vi "Simple Example.vi"() -> ()   [LabVIEW 2020, in "Simple Example.lvlib"]
uses:
  Simple Example.lvlib
  Graphics/Libraries/Raster/Raster.lvlib
  Graphics/Libraries/Raster/Rectangle Dimensions.ctl
  Graphics/Libraries/3D/Camera.ctl
  Graphics/Libraries/3D/3D.lvlib
  Graphics/Libraries/3D/Vector 3D.ctl
  Graphics/Libraries/Utility/Utility.lvlib
  Graphics/Libraries/Raster/UV.ctl
  Graphics/Libraries/3D/Vertex.ctl
  Graphics/Libraries/3D/Triangle.ctl
  7fa56694-391c-4e45-8567-979b4c554bf3.vi
  d55de395-ed50-4187-b237-13a560dfed05.vi
  Graphics/Libraries/Raster/Texture.ctl
  Graphics/Libraries/3D/Material.ctl
panel:
  out "Raaster Time [s]":dbl
  in  "Textured":bool=TRUE
  out "FPS":dbl
  in  "z Transform":sgl(slide)=-15.0 scale=-20.0..10.0
  in  "y Transform":sgl(slide)=5.0 scale=-10.0..10.0
  in  "x Transform":sgl(slide) scale=-10.0..10.0
  in  "z Rotation":sgl(slide) scale=-360.0..360.0
  in  "y Rotation":sgl(slide) scale=-180.0..180.0
  in  "x Rotation":sgl(slide) scale=-360.0..180.0
  out "Screen":picture
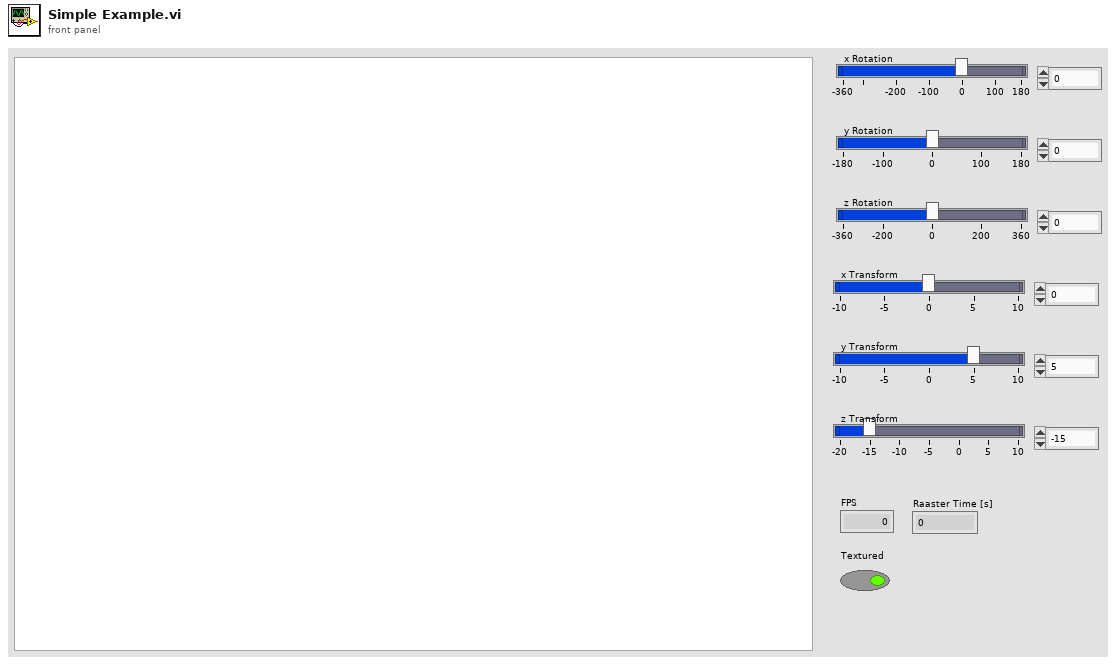
[diagram p1: front panel]
types:
  T1 = typedef "3D.lvlib/Vector 3D.ctl" = cluster{"x":sgl, "y":sgl, "z":sgl}
  T2 = typedef "3D.lvlib/Camera.ctl" = cluster{"Field Of View":sgl, "Near Plane":sgl, "Far Plane":sgl}
  T3 = typedef "Raster.lvlib/Rectangle Dimensions.ctl" = cluster{"Width":u32, "Height":u32}
  T4 = typedef "3D.lvlib/Object.ctl" = cluster{"Triangles":T5[], "Transform":T10, "Name":string, "Alpha Blending Enabled":bool, "Alpha":dbl, "Turntable Enabled":bool, "Material":T8}
  T5 = typedef "3D.lvlib/Triangle.ctl" = cluster{"Vertex 1":T6, "Vertex 2":T6, "Vertex 3":T6, "Alpha":dbl, "Alpha Blending Enabled":bool, "Colour":u32, "Material":T8}
  T6 = typedef "3D.lvlib/Vertex.ctl" = cluster{"Position":T1, "UV":T7, "Colour":u32}
  T7 = typedef "Raster.lvlib/UV.ctl" = cluster{"u":sgl, "v":sgl}
  T8 = typedef "3D.lvlib/Material.ctl" = cluster{"Diffuse Colour":u32, "Texture":T9}
  T9 = typedef "Raster.lvlib/Texture.ctl" = cluster{"Pixels":refnum<data-value>, "Size":T3}
  T10 = typedef "3D.lvlib/Transform.ctl" = cluster{"Position":T1, "Rotation":T1, "Scale":T1}
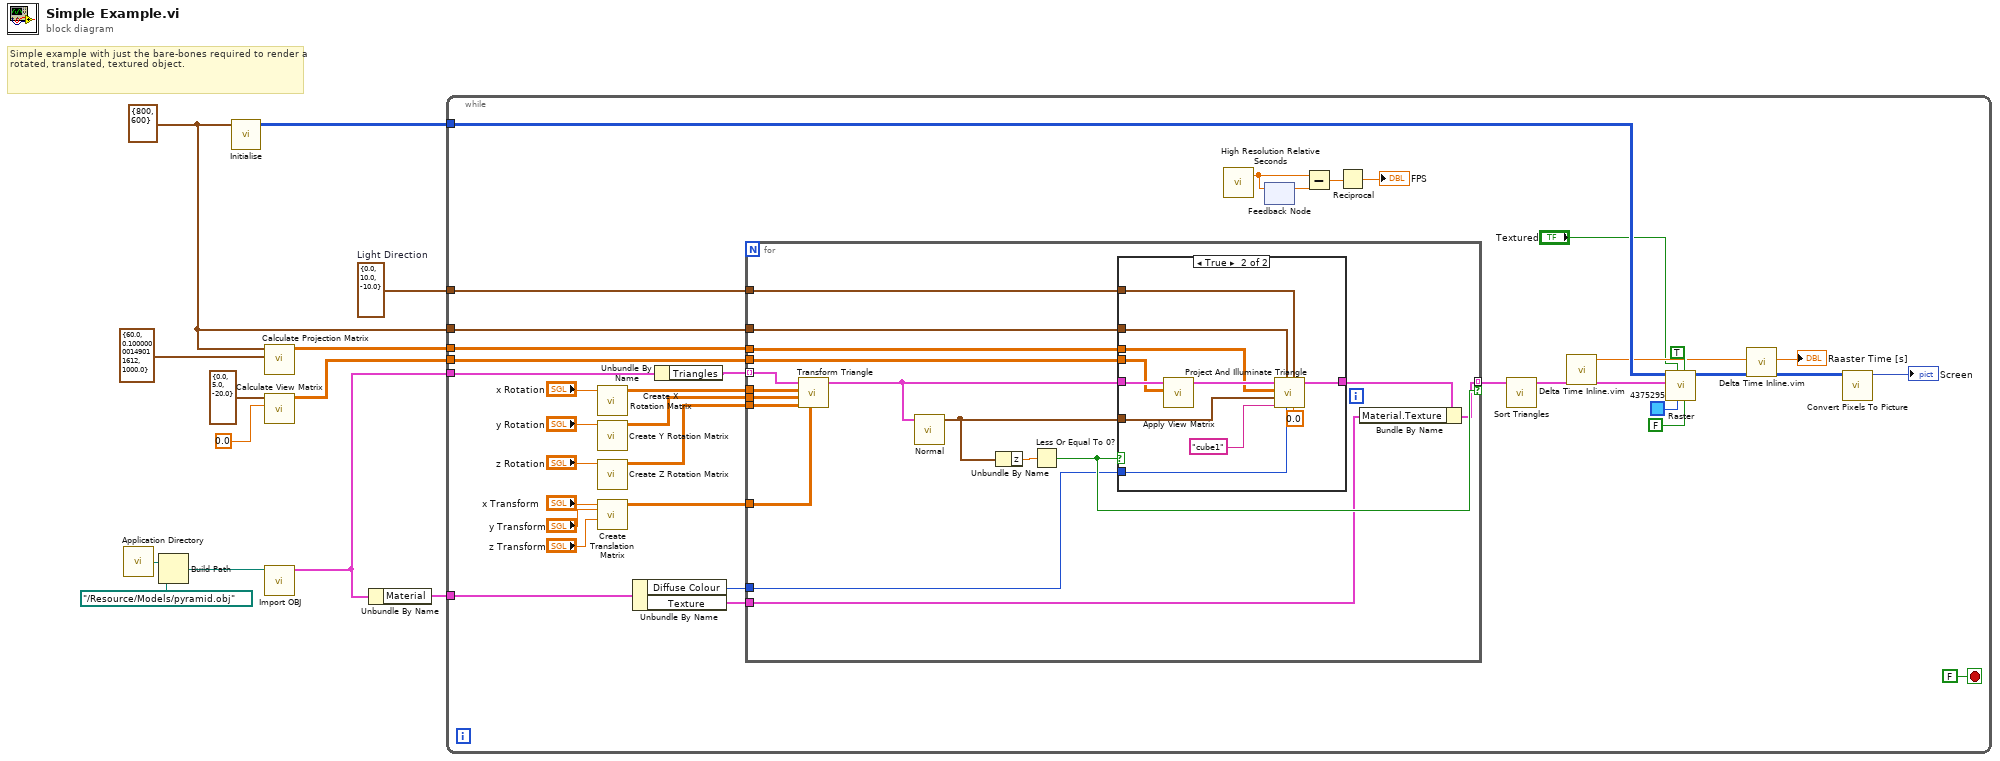
[diagram p0: block diagram]
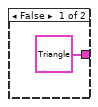
[diagram p2: hidden frame]
diagram:
  w11 = T1 {"x"=0.0, "y"=10.0, "z"=-10.0}  # Light Direction
  w9 = T3 {"Width"=800, "Height"=600} ("Screen Dimensions")
  # "Simple example with just the bare-bones required to render a rotated, translated, textured object."
  n1 = call <vilib>:"Application Directory.vi"() -> ("Application Directory"=w4:path)
  n2 = Build Path(base path=w4, name or relative path=path "../Resource/Models/pyramid.obj") -> (appended path=w3:path)
  n3 = call "Initialise.vi"("Screen Dimensions"=w9) -> ("Pixel Data out"=w8:u32[][])  [unwired: 10 in]
  n4 = call "Calculate Projection Matrix.vi"("Camera"=T2 {"Field Of View"=60.0, "Near Plane"=0.1, "Far Plane"=1000.0}, "Screen Dimensions"=w9) -> ("Projection Matrix"=w10:sgl[][])  [unwired: 9 in]
  n5 = call "Calculate View Matrix.vi"("Camera Rotation"=sgl 0.0, "Camera Position"=T1 {"x"=0.0, "y"=5.0, "z"=-20.0} ("output cluster")) -> ("View Matrix"=w12:sgl[][])  [unwired: 9 in]
  n6 = call "Import OBJ.vi"("Object"=w3) -> ("Object"=w2:T4)  [unwired: 9 in, 1 out]
  n7 = Unbundle By Name(w2) -> ("Material"=w1:T8)
  n8 = while {
    tunnel: w12 -> [w40]
    tunnel: w11 -> [w39]
    tunnel: w10 -> [w38]
    tunnel: w9 -> [w37]
    tunnel: w2 -> [w25]
    tunnel: w8 -> [w36]
    tunnel: w1 -> [w16]
    stop <- FALSE stop-if-true
    n9 = call "Create X Rotation Matrix.vi"("Theta (°)"="x Rotation") -> ("Rotation X Matrix"=w44:sgl[][])  [unwired: 10 in]
    n10 = call "Create Y Rotation Matrix.vi"("Theta (°)"="y Rotation") -> ("Rotation Y Matrix"=w43:sgl[][])  [unwired: 10 in]
    n11 = call "Create Z Rotation Matrix.vi"("Theta (°)"="z Rotation") -> ("Rotation Z Matrix"=w42:sgl[][])  [unwired: 10 in]
    n12 = call "Create Translation Matrix.vi"("z"="z Transform", "y"="y Transform", "x"="x Transform") -> ("Translation Matrix"=w41:sgl[][])  [unwired: 8 in]
    n13 = Unbundle By Name(w16) -> ("Diffuse Colour"=w15:u32, "Texture"=w14:T9)
    n14 = Unbundle By Name(w25) -> ("Triangles"=w26:T5[])
    n15 = for {
      tunnel: w42 -> [w64]
      tunnel: w44 -> [w66]
      tunnel: [w52] -> w24 mode=indexing if=w58
      tunnel: w43 -> [w65]
      tunnel: w41 -> [w63]
      tunnel: w26 -> [w55] mode=indexing
      tunnel: w37 -> [w61]
      tunnel: w38 -> [w60]
      tunnel: w39 -> [w59]
      tunnel: w40 -> [w56]
      tunnel: w15 -> [w54]
      tunnel: w14 -> [w51]
      n16 = call "Transform Triangle.vi"("Translation Matrix"=w63, "Rotation Z Matrix"=w64, "Rotation Y Matrix"=w65, "Rotation X Matrix"=w66, "Triangle in"=w55) -> ("Triangle out"=w62:T5)  [unwired: 6 in]
      n17 = call "Normal.vi"("Triangle"=w62) -> ("Normal"=w67:T1)  [unwired: 10 in]
      n18 = Unbundle By Name(w67) -> ("z"=w57:sgl)
      n19 = Less Or Equal To 0?(x=w57) -> (x <= 0?=w58:bool)
      n20 = case shown="True" w58 {
        tunnel: [T5 {"Vertex 1"={"Position"={"x"=0.0, "y"=0.0, "z"=0.0}, "UV"={"u"=0.0, "v"=0.0}, "Colour"=12517256}, "Vertex 2"={"Position"={"x"=0.0, "y"=0.0, "z"=0.0}, "UV"={"u"=0.0, "v"=0.0}, "Colour"=12517256}, "Vertex 3"={"Position"={"x"=0.0, "y"=0.0, "z"=0.0}, "UV"={"u"=0.0, "v"=0.0}, "Colour"=12517256}, "Alpha"=12517256.0, "Alpha Blending Enabled"=FALSE, "Colour"=0, "Material"={"Diffuse Colour"=0, "Texture"={"Pixels"=refnum, "Size"={"Width"=0, "Height"=0}}}} ("Cluster") w70] -> w53
        tunnel: w67 -> [_ w79]
        tunnel: w62 -> [_ w77]
        tunnel: w61 -> [_ w76]
        tunnel: w60 -> [_ w75]
        tunnel: w59 -> [_ w74]
        tunnel: w56 -> [_ w73]
        tunnel: w54 -> [_ w69]
        frame False {
        }
        frame True {
          n21 = call "Apply View Matrix.vi"("View Matrix"=w73, "Triangle in"=w77) -> ("Triangle out"=w78:T5)  [unwired: 9 in]
          n22 = call "Project And Illuminate Triangle.vi"("Alpha"=0.0, "Light Direction"=w74, "Diffuse Colour"=w69, "Screen Dimensions"=w76, "Name"="cube1", "Normal"=w79, "Projection Matrix"=w75, "Triangle in"=w78) -> ("Triangle out"=w70:T5)  [unwired: 3 in]
        }
      }
      n23 = Bundle By Name(cluster=w53, "Material.Texture"=w51) -> (w52:T5)
    }
    n24 = call <vilib>:"High Resolution Relative Seconds.vi"() -> ("relative seconds"=w30:dbl)
    n25 = feedback-in #1(w30) -> ()
    n26 = feedback #1() -> (w29:dbl)  [unwired: 1 in]
    n27 = Subtract(x=w30, y=w29) -> (x-y=w28:dbl)
    n28 = Reciprocal(x=w28) -> (1/x=→"FPS":dbl)
    n29 = call "Sort Triangles.vi"("Triangles"=w24) -> ("Triangles Sorted"=w23:T5[])  [unwired: 10 in]
    n30 = call "Delta Time Inline.vim"("value in"=w23) -> ("value out"=w22:T5[], "Relative Seconds out [s]"=w19:dbl)  [unwired: 8 in, 1 out]
    n31 = call "Raster.vi"("Draw Lines"=FALSE, "Draw Triangles"=TRUE, "Line Colour"=u32 4375295, "Textured"="Textured", "Triangles Sorted"=w22, "Pixel Data in"=w36) -> ("Pixel Data out"=w21:u32[][])  [unwired: 5 in]
    n32 = call "Delta Time Inline.vim"("value in"=w21, "Relative Seconds in [s]"=w19) -> ("value out"=w20:u32[][], "Delta Time [s]"=→"Raaster Time [s]":dbl)  [unwired: 7 in, 1 out]
    n33 = call "Convert Pixels To Picture.vi"("Pixel Data in"=w20) -> ("2D Picture"=→"Screen":picture)  [unwired: 9 in, 1 out]
  }
